vi "Distribution Plot.vi"() -> (0 "Distribution Plot":picture)   [LabVIEW 2012]
uses:
  <vilib>/picture/cartesn2.llb/XY Plot Type.ctl
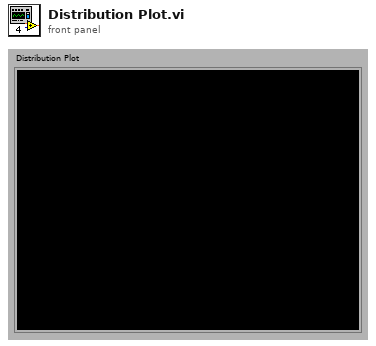
[diagram p1: front panel]
types:
  T1 = typedef "XY Plot Type.ctl" = enum16{"points", "squares", "circles", "connected points", "connected squares", "connected circles", "comb plot", "sized scatter plot", "sized-colored scatter plot", "min-max lines"}
  T2 = cluster{"plot color":u32, "xy plot type":T1, "baseline":dbl}
  T3 = cluster{"line color":u32, "text color":u32, "tick length":i16, "crossing axes":bool, "visible grid?":bool}
  T4 = typedef "LVBoundsTypeDef.ctl" = cluster{"Width":u32, "Height":u32}
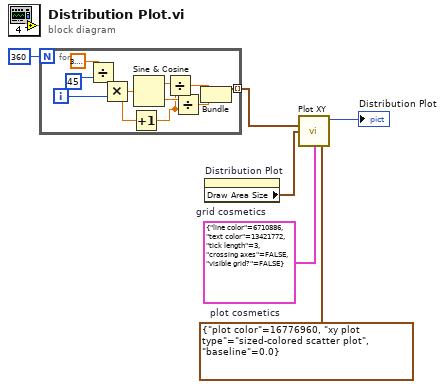
[diagram p0: block diagram]
diagram:
  w5 = T2 {"plot color"=16776960, "xy plot type"=enum."sized-colored scatter plot", "baseline"=0.0}  # plot cosmetics
  w6 = T3 {"line color"=6710886, "text color"=13421772, "tick length"=3, "crossing axes"=FALSE, "visible grid?"=FALSE}  # grid cosmetics
  n1 = for {
    N: 360 -> [_]
    tunnel: [w16] -> w1 mode=indexing
    i -> [w7]
    n2 = Divide(x=3.141592653589793, y=45) -> (x/y=w17:dbl)
    n3 = Multiply(x=w17, y=w7) -> (x*y=w9:dbl)
    n4 = Increment(x=w9) -> (x+1=w8:dbl)
    n5 = Sine & Cosine(0:w9) -> (1:w13:dbl, 2:w11:dbl)
    n6 = Divide(x=w13, y=w8) -> (x/y=w12:dbl)
    n7 = Divide(x=w11, y=w8) -> (x/y=w10:dbl)
    n8 = Bundle(w12, w10) -> (w16:cluster{dbl, dbl})  [unwired: 1 out]
  }
  n9 = property on="Distribution Plot" class="Pict"() -> ("Draw Area Size"=w4:T4)  [unwired: 2 in, 2 out]
  n10 = call <vilib>:"Plot XY.vi"("data"=w1, "dimensions (w,h)"=w4, "cartesian grid cosmetics"=w6, "XY plot cosmetics"=w5) -> ("new picture"=→"Distribution Plot":picture)  [unwired: 2 in, 9 out]
